vi "Test Apply Filter to Log Data.vi"(8 "error in (no error)":errorcluster, 11 "Test Case In":refnum<class "Debug Log Test.lvclass">) -> (0 "error out":errorcluster, 3 "Test Case Out":refnum<class "Debug Log Test.lvclass">)   [LabVIEW 2020, in "Debug Log Test.lvclass"]
uses:
  Debug Log Test.lvclass
  C:/Program Files (x86)/National Instruments/LabVIEW 2020/vi.lib/Astemes/LUnit/Test Case.lvclass
  source/Debug Log/Debug Log.lvclass
  source/Debug Log/Debug Log.lvclass/Debug Log.ctl
  <vilib>/Astemes/LUnit/Test Case.lvclass/Test Case.ctl
  <vilib>/Astemes/LUnit/LUnit Assertion Result.lvclass/LUnit Assertion Result.ctl
  <vilib>/Astemes/LUnit/LUnit Test Case Result.lvclass/LUnit Test Case Result.ctl
  <vilib>/Astemes/LUnit/LUnit Method Result.lvclass/LUnit Method Result.ctl
  01074fa8-ee8a-411d-bc8b-fc92c4f90959.vi
  source/Debug Log/Read Unfiltered Log Content.vi
  <vilib>/Astemes/LUnit/Palette/Pass.vi
  <vilib>/Astemes/LUnit/Palette/Fail.vi
  <vilib>/Astemes/LUnit/Compare Variants.vi
  <vilib>/Astemes/LUnit/Describe Comparison.vi
  <vilib>/Astemes/LUnit/Set Assertion Type.vi
  <vilib>/Astemes/LUnit/Add test result.vi
  <vilib>/Astemes/LUnit/LUnit Write Passed.vi
  <vilib>/Astemes/LUnit/LUnit Write Message.vi
  <vilib>/Astemes/LUnit/LUnit Write Description.vi
  <vilib>/Astemes/LUnit/Variant to string.vi
  <vilib>/Astemes/LUnit/LUnit Write Assertion Type.vi
  <vilib>/Astemes/LUnit/LUnit Record Assertion Result.vi
  <vilib>/Astemes/LUnit/LUnit Aggregate Assertion Results.vi
  <vilib>/Astemes/LUnit/Assertion Result/LUnit Read Status.vi
  <vilib>/Astemes/LUnit/LUnit Read Message.vi
  <vilib>/Astemes/LUnit/LUnit Read Description.vi
  <vilib>/Astemes/LUnit/Method Result/LUnit Merge Status.vi
  <vilib>/Astemes/LUnit/LUnit Concatenate result strings.vi
  source/Mock Filter/Mock Filter.lvclass
  C:/Users/anton/Documents/GitHub/triarc-debugger/source/Filter/Filter.lvclass
  <vilib>/Utility/Data Type/Get Type Information.vi
  <vilib>/Utility/LVClass/Get LV Class Name.vi
  <vilib>/Astemes/LUnit/LUnit Assertion Result.lvclass
  source/Filter/Filter.lvclass
  Debug Log Test.lvclass/Debug Log Test.ctl
  source/Debug Data/Debug Data.lvclass
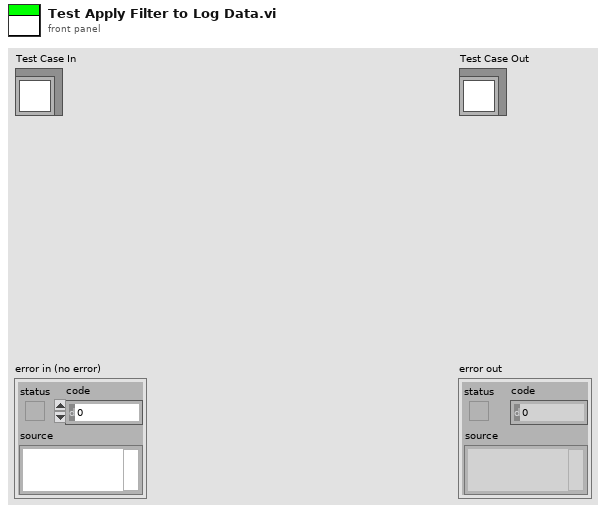
[diagram p1: front panel]
types:
  T1 = cluster{"Action":string, "Call Chain":string, "Process":string, "Message":string, "Message Data":variant, "Time":dbl}[]
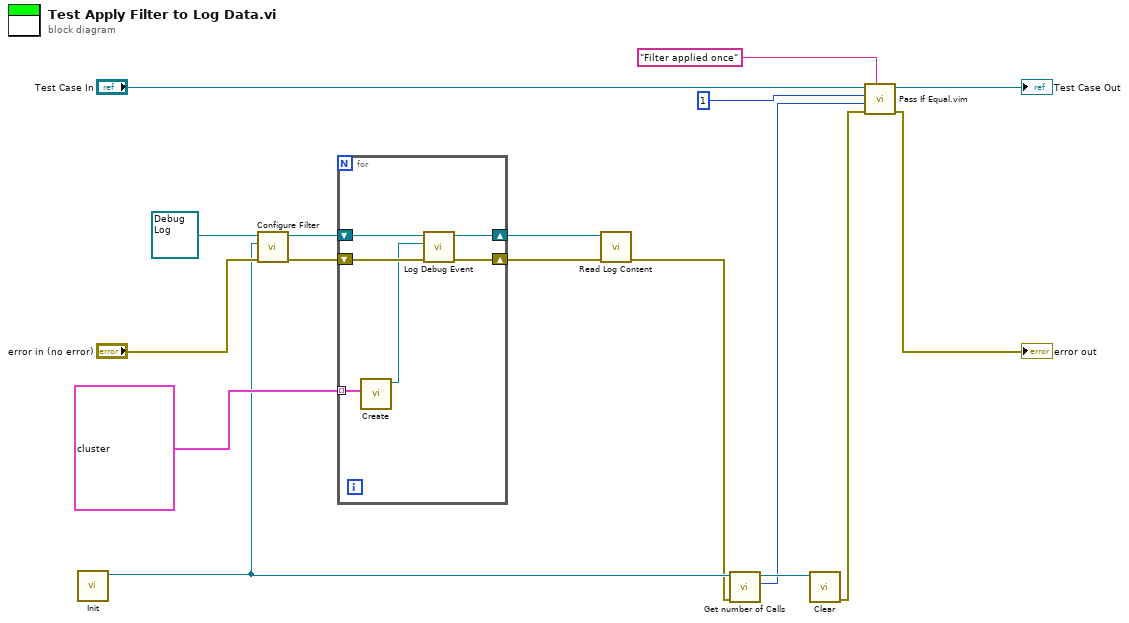
[diagram p0: block diagram]
diagram:
  n1 = call "Init.vi"() -> ("Mock Filter out"=w5:refnum<class "Mock Filter.lvclass">)  [unwired: 10 in, 1 out]
  n2 = call "Configure Filter.vi"("error in (no error)"="error in (no error)", "Filter"=w5, "Debug Log In"=refnum<class "Debug Log.lvclass"> refnum ("Debug Log.lvclass")) -> ("error out"=w8:errorcluster, "Debug Log Out"=w6:refnum<class "Debug Log.lvclass">)  [unwired: 7 in]
  n3 = for {
    tunnel: T1 [{"Action"="", "Call Chain"="", "Process"="", "Message"="1", "Message Data"=variant, "Time"=0.0}, {"Action"="", "Call Chain"="", "Process"="", "Message"="2", "Message Data"=variant, "Time"=0.0}, {"Action"="", "Call Chain"="", "Process"="", "Message"="3", "Message Data"=variant, "Time"=0.0}] ("Debug Data Cluster") -> [w19] mode=indexing
    shift-right: [w22] -> w9
    shift-left: w6 -> [w23]
    shift-right: [w20] -> w15
    shift-left: w8 -> [w21]
    n4 = call "Create.vi"("Debug Data Cluster"=w19) -> ("Debug Data out"=w18:refnum<class "Debug Data.lvclass">)  [unwired: 9 in, 1 out]
    n5 = call "Log Debug Event.vi"("error in (no error)"=w21, "Debug Data.lvclass"=w18, "Debugger in"=w23) -> ("error out"=w20:errorcluster, "Debugger out"=w22:refnum<class "Debug Log.lvclass">)  [unwired: 7 in]
  }
  n6 = call "Read Log Content.vi"("error in (no error)"=w15, "Debug Log In"=w9) -> ("error out"=w2:errorcluster)  [unwired: 7 in, 2 out]
  n7 = call "Get number of Calls.vi"("error in (no error)"=w2, "Mock Filter in"=w5) -> ("Number of Calls"=w3:i32, "Mock Filter out"=w4:refnum<class "Mock Filter.lvclass">)  [unwired: 7 in, 1 out]
  n8 = call "Clear.vi"("Mock Filter in"=w4) -> ("error out"=w1:errorcluster)  [unwired: 9 in, 1 out]
  n9 = call "Pass If Equal.vim"("Description"="Filter applied once", "error in (no error)"=w1, "Actual"=w3, "Expected"=1 ("size(s)"), "LUnit Test Case In"="Test Case In") -> ("error out"=→"error out":errorcluster, "LUnit Test Case Out"=→"Test Case Out":refnum<class "Debug Log Test.lvclass">)  [unwired: 5 in]
